vi "API_Calculate_Time.vi"(1 "Time":dbl, 2 "Argument List In":string[](array[string])) -> (0 "Argument List Out":string[](array[string]))   [LabVIEW 2011]
doc: "This VI, when called within an API event, will set the \"Time\" parameter in the Growth Sequence Editor to the given input value."
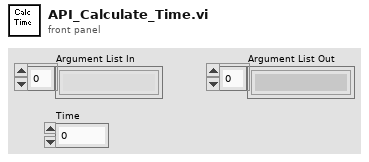
[diagram p1: front panel]
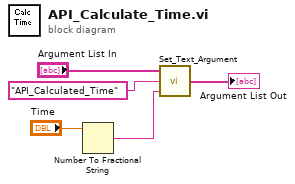
[diagram p0: block diagram]
diagram:
  n1 = Number To Fractional String(number="Time") -> (F-format string=w2:string)  [unwired: 3 in]
  n2 = call "Set_Text_Argument.vi"("Text"=w2, "Argument"="API_Calculated_Time", "Argument List In"="Argument List In") -> ("Argument List Out"=→"Argument List Out":string[])
